vi "unpack tcp packet.vi"(11 "TCP Pack":string="\u0000resp      啊手动阀手动阀") -> (2 "tcp-message-type":T1=enum."resp", 3 "String":string="啊手动阀手动阀")   [LabVIEW 2020, in "CSM-TCP-Router.lvlib"]
uses:
  CSM-TCP-Router.lvlib
  typedef/tcp-msg type.ctl
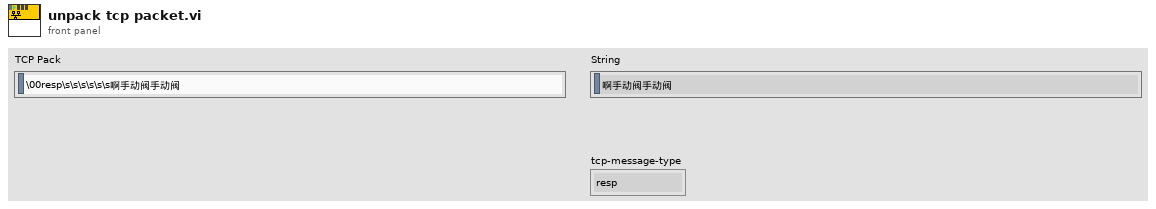
[diagram p1: front panel]
types:
  T1 = typedef "CSM-TCP-Router.lvlib/tcp-msg type.ctl" = enum8{"info", "error", "cmd", "resp", "async-resp", "status", "interrupt"}
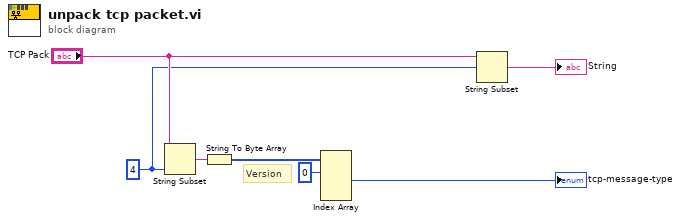
[diagram p0: block diagram]
diagram:
  w2 = 4 ("length (rest)")
  # "Version"
  n1 = String Subset(string="TCP Pack", length (rest)=w2) -> (substring=w7:string)  [unwired: 1 in]
  n2 = String To Byte Array(string=w7) -> (unsigned byte array=w6:u8[])
  n3 = Index Array(array=w6, index #1=0 ("index")) -> (element #2=→"tcp-message-type":u8)  [unwired: 3 in, 3 out]
  n4 = String Subset(string="TCP Pack", offset (0)=w2) -> (substring=→"String":string)  [unwired: 1 in]
